vi "Update Test Server.vi"(8 "error in (no error)":errorcluster, 10 "Lines":T2[](array[typedef]) {"OPC UA Data Type" items=["Boolean"=1, "SByte"=2, "Byte"=3, "Int16"=4, "UInt16"=5, "Int32"=6, "UInt32"=7, "Int64"=8, "UInt64"=9, "Float"=10, "Double"=11, "String"=12, "DateTime"=13, "ByteString"=15, "Array of Boolean"=101, "Array of SByte"=102, "Array of Byte"=103, "Array of Int16"=104, "Array of UInt16"=105, "Array of Int32"=106, "Array of UInt32"=107, "Array of Int64"=108, "Array of UInt64"=109, "Array of Float"=110, "Array of Double"=111, "Array of String"=112, "Array of DateTime"=113, "Array of ByteString"=115]}, 11 "OPC UA server refnum in":refnum<k21>) -> (0 "error out":errorcluster, 2 "Server Data":T1(array[cluster]))   [LabVIEW 2013, in "OPC UA Client Tests.lvlib"]
doc: "Forces the OPC UA server to update every line in given configuration. Passes out cluster of node paths and flattened data to be compared to tag bus."
uses:
  OPC UA Client Tests.lvlib
  module/configuration/Line.ctl
  <vilib>/NI/Tag Bus Module Framework/channel/TBM channel.lvclass
  module/configuration/OPC UA Data Type.ctl
  <vilib>/OPCUA/server/Write Bool.vi
  <vilib>/OPCUA/server/Write SByte.vi
  <vilib>/OPCUA/server/Write Byte.vi
  <vilib>/OPCUA/server/Write Int16.vi
  <vilib>/OPCUA/server/Write UInt16.vi
  <vilib>/OPCUA/server/Write Int32.vi
  <vilib>/OPCUA/server/Write UInt32.vi
  <vilib>/OPCUA/server/Write Int64.vi
  <vilib>/OPCUA/server/Write UInt64.vi
  <vilib>/OPCUA/server/Write Float.vi
  <vilib>/OPCUA/server/Write Double.vi
  <vilib>/OPCUA/server/Write String.vi
  <vilib>/OPCUA/server/Write Date Time.vi
  <vilib>/OPCUA/server/Write Byte String.vi
  <vilib>/OPCUA/server/Write Bool Array.vi
  <vilib>/OPCUA/server/Write SByte Array.vi
  <vilib>/OPCUA/server/Write Byte Array.vi
  <vilib>/OPCUA/server/Write Int16 Array.vi
  <vilib>/OPCUA/server/Write UInt16 Array.vi
  <vilib>/OPCUA/server/Write Int32 Array.vi
  <vilib>/OPCUA/server/Write UInt32 Array.vi
  <vilib>/OPCUA/server/Write Int64 Array.vi
  <vilib>/OPCUA/server/Write UInt64 Array.vi
  <vilib>/OPCUA/server/Write Float Array.vi
  <vilib>/OPCUA/server/Write Double Array.vi
  <vilib>/OPCUA/server/Write String Array.vi
  <vilib>/OPCUA/server/Write Date Time Array.vi
  <vilib>/opcua/NI OPC UA Server.lvlib
  module/configuration/OPC UA Client configuration.lvclass
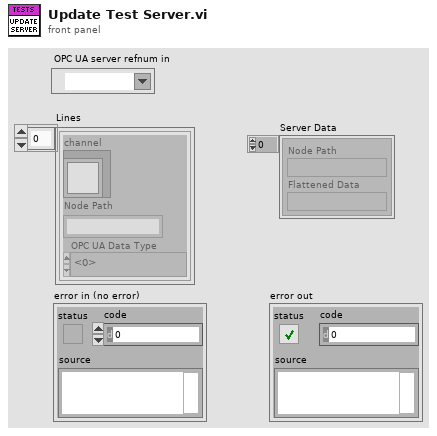
[diagram p1: front panel]
types:
  T1 = cluster{"Node Path":string, "Flattened Data":string}[]
  T2 = typedef "OPC UA Client configuration.lvclass/Line.ctl" = cluster{"channel":refnum<class "TBM channel.lvclass">, "Node Path":string, "OPC UA Data Type":T3}
  T3 = typedef "OPC UA Client configuration.lvclass/OPC UA Data Type.ctl" = u16
  T4 = cluster{"Node Path":string, "Flattened Data":string}
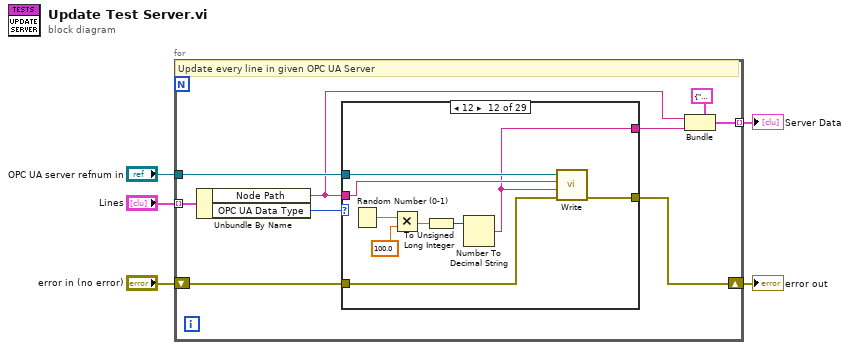
[diagram p0: block diagram]
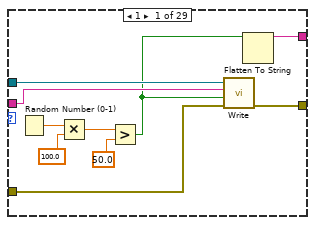
[diagram p2: hidden frame]
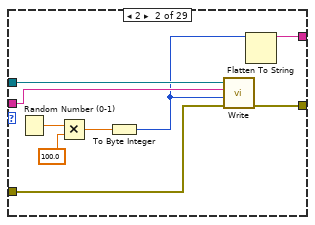
[diagram p3: hidden frame]
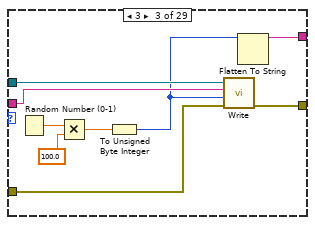
[diagram p4: hidden frame]
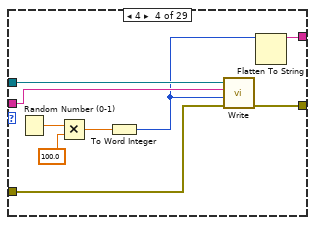
[diagram p5: hidden frame]
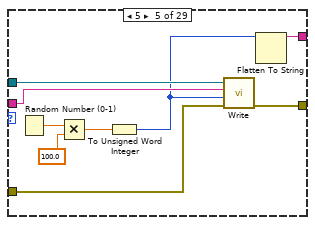
[diagram p6: hidden frame]
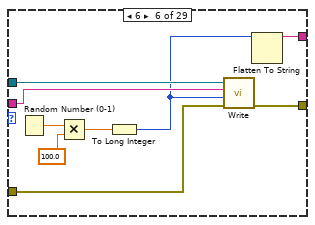
[diagram p7: hidden frame]
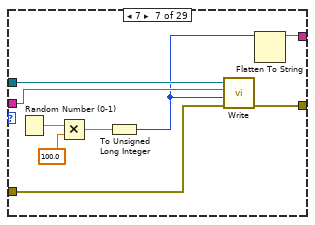
[diagram p8: hidden frame]
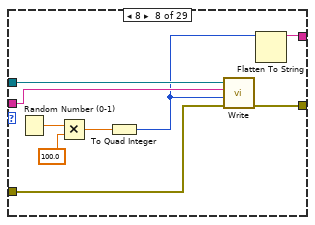
[diagram p9: hidden frame]
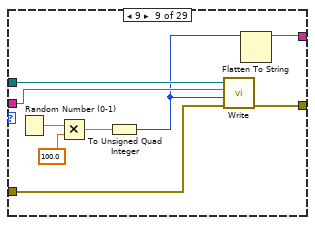
[diagram p10: hidden frame]
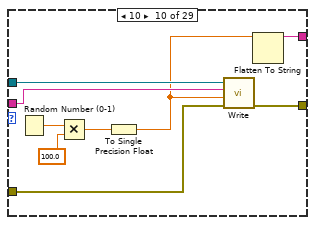
[diagram p11: hidden frame]
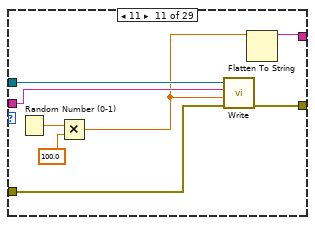
[diagram p12: hidden frame]
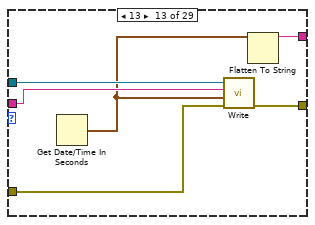
[diagram p13: hidden frame]
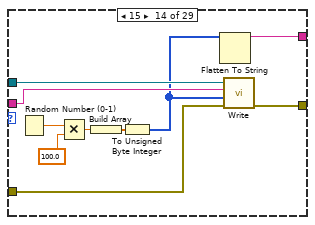
[diagram p14: hidden frame]
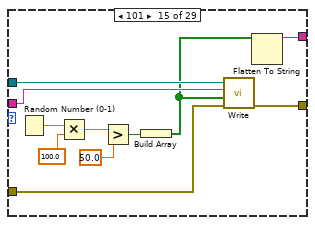
[diagram p15: hidden frame]
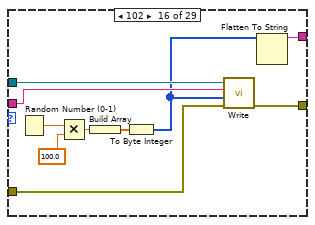
[diagram p16: hidden frame]
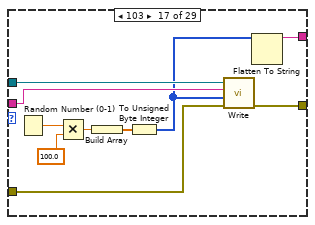
[diagram p17: hidden frame]
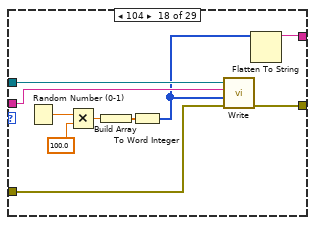
[diagram p18: hidden frame]
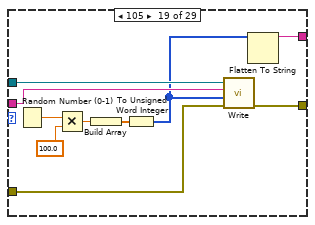
[diagram p19: hidden frame]
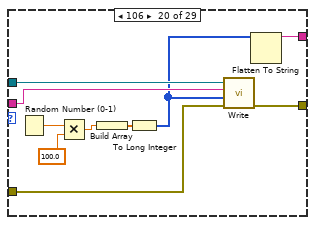
[diagram p20: hidden frame]
diagram:
  n1 = for {
    tunnel: "OPC UA server refnum in" -> [w14]
    tunnel: "Lines" -> [w13] mode=indexing
    tunnel: [w6] -> w1 mode=indexing
    shift-right: [w10] -> w3
    shift-left: "error in (no error)" -> [w11]
    # "Update every line in given OPC UA Server"
    n2 = Unbundle By Name(w13) -> ("Node Path"=w7:string, "OPC UA Data Type"=w12:T3)
    n3 = case shown="12" w12 {
      tunnel: w14 -> [w24 w33 w42 w51 w60 w69 w78 w87 w96 w105 w113 w122 w128 w138 w149 w159 w169 w179 w189 w199 w209 w219 w229 w239 w248 w258 w265 w275 _]
      tunnel: w7 -> [w23 w32 w41 w50 w59 w68 w77 w86 w95 w104 w112 w121 w127 w137 w148 w158 w168 w178 w188 w198 w208 w218 w228 w238 w247 w257 w264 w274 _]
      tunnel: w11 -> [w22 w31 w40 w49 w58 w67 w76 w85 w94 w103 w111 w120 w126 w136 w147 w157 w167 w177 w187 w197 w207 w217 w227 w237 w246 w256 w263 w273 _]
      tunnel: [w21 w30 w39 w48 w57 w66 w75 w84 w93 w102 w110 w119 w125 w135 w146 w156 w166 w176 w186 w196 w206 w216 w226 w236 w245 w255 w262 w272 errorcluster {"status"=TRUE, "code"=0, "source"="Invalid UA Data Type"} ("error out")] -> w10
      tunnel: [w15 w27 w35 w44 w54 w63 w72 w81 w90 w98 w107 w115 w124 w129 w140 w151 w162 w172 w182 w192 w202 w212 w222 w231 w241 w250 w260 w267 "" ("data string")] -> w9
      frame 1 {
        n4 = Random Number (0-1)() -> (number: 0 to 1=w20:dbl)
        n5 = Multiply(x=w20, y=100.0) -> (x*y=w18:dbl)
        n6 = Greater?(x=w18, y=50.0) -> (0:w16:bool)
        n7 = call-poly <vilib>:"Write.vi"("error in (no error)"=w22, "value"=w16, "node path"=w23, "OPC UA server refnum in"=w24) -> ("error out"=w21:errorcluster)  [unwired: 6 in, 1 out]
        n8 = Flatten To String(anything=w16) -> (data string=w15:string)  [unwired: 3 in, 2 out]
      }
      frame 2 {
        n9 = Random Number (0-1)() -> (number: 0 to 1=w29:dbl)
        n10 = Multiply(x=w29, y=100.0) -> (x*y=w26:dbl)
        n11 = To Byte Integer(number=w26) -> (8bit integer=w25:i8)
        n12 = call-poly <vilib>:"Write.vi"("error in (no error)"=w31, "value"=w25, "node path"=w32, "OPC UA server refnum in"=w33) -> ("error out"=w30:errorcluster)  [unwired: 6 in, 1 out]
        n13 = Flatten To String(anything=w25) -> (data string=w27:string)  [unwired: 3 in, 2 out]
      }
      frame 3 {
        n14 = Random Number (0-1)() -> (number: 0 to 1=w38:dbl)
        n15 = Multiply(x=w38, y=100.0) -> (x*y=w36:dbl)
        n16 = To Unsigned Byte Integer(number=w36) -> (unsigned 8bit integer=w34:u8)
        n17 = call-poly <vilib>:"Write.vi"("error in (no error)"=w40, "value"=w34, "node path"=w41, "OPC UA server refnum in"=w42) -> ("error out"=w39:errorcluster)  [unwired: 6 in, 1 out]
        n18 = Flatten To String(anything=w34) -> (data string=w35:string)  [unwired: 3 in, 2 out]
      }
      frame 4 {
        n19 = Random Number (0-1)() -> (number: 0 to 1=w47:dbl)
        n20 = Multiply(x=w47, y=100.0) -> (x*y=w45:dbl)
        n21 = To Word Integer(number=w45) -> (16bit integer=w43:i16)
        n22 = call-poly <vilib>:"Write.vi"("error in (no error)"=w49, "value"=w43, "node path"=w50, "OPC UA server refnum in"=w51) -> ("error out"=w48:errorcluster)  [unwired: 6 in, 1 out]
        n23 = Flatten To String(anything=w43) -> (data string=w44:string)  [unwired: 3 in, 2 out]
      }
      frame 5 {
        n24 = Random Number (0-1)() -> (number: 0 to 1=w56:dbl)
        n25 = Multiply(x=w56, y=100.0) -> (x*y=w53:dbl)
        n26 = To Unsigned Word Integer(number=w53) -> (unsigned 16bit integer=w52:u16)
        n27 = call-poly <vilib>:"Write.vi"("error in (no error)"=w58, "value"=w52, "node path"=w59, "OPC UA server refnum in"=w60) -> ("error out"=w57:errorcluster)  [unwired: 6 in, 1 out]
        n28 = Flatten To String(anything=w52) -> (data string=w54:string)  [unwired: 3 in, 2 out]
      }
      frame 6 {
        n29 = Random Number (0-1)() -> (number: 0 to 1=w65:dbl)
        n30 = Multiply(x=w65, y=100.0) -> (x*y=w62:dbl)
        n31 = To Long Integer(number=w62) -> (32bit integer=w61:i32)
        n32 = call-poly <vilib>:"Write.vi"("error in (no error)"=w67, "value"=w61, "node path"=w68, "OPC UA server refnum in"=w69) -> ("error out"=w66:errorcluster)  [unwired: 6 in, 1 out]
        n33 = Flatten To String(anything=w61) -> (data string=w63:string)  [unwired: 3 in, 2 out]
      }
      frame 7 {
        n34 = Random Number (0-1)() -> (number: 0 to 1=w74:dbl)
        n35 = Multiply(x=w74, y=100.0) -> (x*y=w71:dbl)
        n36 = To Unsigned Long Integer(number=w71) -> (unsigned 32bit integer=w70:u32)
        n37 = call-poly <vilib>:"Write.vi"("error in (no error)"=w76, "value"=w70, "node path"=w77, "OPC UA server refnum in"=w78) -> ("error out"=w75:errorcluster)  [unwired: 6 in, 1 out]
        n38 = Flatten To String(anything=w70) -> (data string=w72:string)  [unwired: 3 in, 2 out]
      }
      frame 8 {
        n39 = Random Number (0-1)() -> (number: 0 to 1=w83:dbl)
        n40 = Multiply(x=w83, y=100.0) -> (x*y=w80:dbl)
        n41 = To Quad Integer(1:w80) -> (0:w79:i64)
        n42 = call-poly <vilib>:"Write.vi"("error in (no error)"=w85, "value"=w79, "node path"=w86, "OPC UA server refnum in"=w87) -> ("error out"=w84:errorcluster)  [unwired: 6 in, 1 out]
        n43 = Flatten To String(anything=w79) -> (data string=w81:string)  [unwired: 3 in, 2 out]
      }
      frame 9 {
        n44 = Random Number (0-1)() -> (number: 0 to 1=w92:dbl)
        n45 = Multiply(x=w92, y=100.0) -> (x*y=w89:dbl)
        n46 = To Unsigned Quad Integer(1:w89) -> (0:w88:u64)
        n47 = call-poly <vilib>:"Write.vi"("error in (no error)"=w94, "value"=w88, "node path"=w95, "OPC UA server refnum in"=w96) -> ("error out"=w93:errorcluster)  [unwired: 6 in, 1 out]
        n48 = Flatten To String(anything=w88) -> (data string=w90:string)  [unwired: 3 in, 2 out]
      }
      frame 10 {
        n49 = Random Number (0-1)() -> (number: 0 to 1=w101:dbl)
        n50 = Multiply(x=w101, y=100.0) -> (x*y=w99:dbl)
        n51 = To Single Precision Float(number=w99) -> (single precision float=w97:sgl)
        n52 = call-poly <vilib>:"Write.vi"("error in (no error)"=w103, "value"=w97, "node path"=w104, "OPC UA server refnum in"=w105) -> ("error out"=w102:errorcluster)  [unwired: 6 in, 1 out]
        n53 = Flatten To String(anything=w97) -> (data string=w98:string)  [unwired: 3 in, 2 out]
      }
      frame 11 {
        n54 = Random Number (0-1)() -> (number: 0 to 1=w109:dbl)
        n55 = Multiply(x=w109, y=100.0) -> (x*y=w106:dbl)
        n56 = call-poly <vilib>:"Write.vi"("error in (no error)"=w111, "value"=w106, "node path"=w112, "OPC UA server refnum in"=w113) -> ("error out"=w110:errorcluster)  [unwired: 6 in, 1 out]
        n57 = Flatten To String(anything=w106) -> (data string=w107:string)  [unwired: 3 in, 2 out]
      }
      frame 12 {
        n58 = Random Number (0-1)() -> (number: 0 to 1=w118:dbl)
        n59 = Multiply(x=w118, y=100.0) -> (x*y=w116:dbl)
        n60 = To Unsigned Long Integer(number=w116) -> (unsigned 32bit integer=w114:u32)
        n61 = Number To Decimal String(number=w114) -> (decimal integer string=w115:string)  [unwired: 1 in]
        n62 = call-poly <vilib>:"Write.vi"("error in (no error)"=w120, "value"=w115, "node path"=w121, "OPC UA server refnum in"=w122) -> ("error out"=w119:errorcluster)  [unwired: 6 in, 1 out]
      }
      frame 13 {
        n63 = Get Date/Time In Seconds() -> (seconds since 1Jan1904=w123:timestamp)
        n64 = call-poly <vilib>:"Write.vi"("error in (no error)"=w126, "value"=w123, "node path"=w127, "OPC UA server refnum in"=w128) -> ("error out"=w125:errorcluster)  [unwired: 6 in, 1 out]
        n65 = Flatten To String(anything=w123) -> (data string=w124:string)  [unwired: 3 in, 2 out]
      }
      frame 15 {
        n66 = Random Number (0-1)() -> (number: 0 to 1=w134:dbl)
        n67 = Multiply(x=w134, y=100.0) -> (x*y=w132:dbl)
        n68 = Build Array(w132) -> (w131:dbl[])
        n69 = To Unsigned Byte Integer(number=w131) -> (unsigned 8bit integer=w130:u8[])
        n70 = Flatten To String(anything=w130) -> (data string=w129:string)  [unwired: 3 in, 2 out]
        n71 = call-poly <vilib>:"Write.vi"("error in (no error)"=w136, "value"=w130, "node path"=w137, "OPC UA server refnum in"=w138) -> ("error out"=w135:errorcluster)  [unwired: 6 in, 1 out]
      }
      frame 101 {
        n72 = Random Number (0-1)() -> (number: 0 to 1=w145:dbl)
        n73 = Multiply(x=w145, y=100.0) -> (x*y=w143:dbl)
        n74 = Greater?(x=w143, y=50.0) -> (0:w141:bool)
        n75 = Build Array(w141) -> (w139:bool[])
        n76 = call-poly <vilib>:"Write.vi"("error in (no error)"=w147, "value"=w139, "node path"=w148, "OPC UA server refnum in"=w149) -> ("error out"=w146:errorcluster)  [unwired: 6 in, 1 out]
        n77 = Flatten To String(anything=w139) -> (data string=w140:string)  [unwired: 3 in, 2 out]
      }
      frame 102 {
        n78 = Random Number (0-1)() -> (number: 0 to 1=w155:dbl)
        n79 = Multiply(x=w155, y=100.0) -> (x*y=w153:dbl)
        n80 = Build Array(w153) -> (w152:dbl[])
        n81 = To Byte Integer(number=w152) -> (8bit integer=w150:i8[])
        n82 = call-poly <vilib>:"Write.vi"("error in (no error)"=w157, "value"=w150, "node path"=w158, "OPC UA server refnum in"=w159) -> ("error out"=w156:errorcluster)  [unwired: 6 in, 1 out]
        n83 = Flatten To String(anything=w150) -> (data string=w151:string)  [unwired: 3 in, 2 out]
      }
      frame 103 {
        n84 = Random Number (0-1)() -> (number: 0 to 1=w165:dbl)
        n85 = Multiply(x=w165, y=100.0) -> (x*y=w163:dbl)
        n86 = Build Array(w163) -> (w161:dbl[])
        n87 = To Unsigned Byte Integer(number=w161) -> (unsigned 8bit integer=w160:u8[])
        n88 = call-poly <vilib>:"Write.vi"("error in (no error)"=w167, "value"=w160, "node path"=w168, "OPC UA server refnum in"=w169) -> ("error out"=w166:errorcluster)  [unwired: 6 in, 1 out]
        n89 = Flatten To String(anything=w160) -> (data string=w162:string)  [unwired: 3 in, 2 out]
      }
      frame 104 {
        n90 = Random Number (0-1)() -> (number: 0 to 1=w175:dbl)
        n91 = Multiply(x=w175, y=100.0) -> (x*y=w173:dbl)
        n92 = Build Array(w173) -> (w171:dbl[])
        n93 = To Word Integer(number=w171) -> (16bit integer=w170:i16[])
        n94 = call-poly <vilib>:"Write.vi"("error in (no error)"=w177, "value"=w170, "node path"=w178, "OPC UA server refnum in"=w179) -> ("error out"=w176:errorcluster)  [unwired: 6 in, 1 out]
        n95 = Flatten To String(anything=w170) -> (data string=w172:string)  [unwired: 3 in, 2 out]
      }
      frame 105 {
        n96 = Random Number (0-1)() -> (number: 0 to 1=w185:dbl)
        n97 = Multiply(x=w185, y=100.0) -> (x*y=w183:dbl)
        n98 = Build Array(w183) -> (w181:dbl[])
        n99 = To Unsigned Word Integer(number=w181) -> (unsigned 16bit integer=w180:u16[])
        n100 = call-poly <vilib>:"Write.vi"("error in (no error)"=w187, "value"=w180, "node path"=w188, "OPC UA server refnum in"=w189) -> ("error out"=w186:errorcluster)  [unwired: 6 in, 1 out]
        n101 = Flatten To String(anything=w180) -> (data string=w182:string)  [unwired: 3 in, 2 out]
      }
      frame 106 {
        n102 = Random Number (0-1)() -> (number: 0 to 1=w195:dbl)
        n103 = Multiply(x=w195, y=100.0) -> (x*y=w193:dbl)
        n104 = Build Array(w193) -> (w191:dbl[])
        n105 = To Long Integer(number=w191) -> (32bit integer=w190:i32[])
        n106 = call-poly <vilib>:"Write.vi"("error in (no error)"=w197, "value"=w190, "node path"=w198, "OPC UA server refnum in"=w199) -> ("error out"=w196:errorcluster)  [unwired: 6 in, 1 out]
        n107 = Flatten To String(anything=w190) -> (data string=w192:string)  [unwired: 3 in, 2 out]
      }
      frame 107 {
        n108 = Random Number (0-1)() -> (number: 0 to 1=w205:dbl)
        n109 = Multiply(x=w205, y=100.0) -> (x*y=w203:dbl)
        n110 = Build Array(w203) -> (w201:dbl[])
        n111 = To Unsigned Long Integer(number=w201) -> (unsigned 32bit integer=w200:u32[])
        n112 = call-poly <vilib>:"Write.vi"("error in (no error)"=w207, "value"=w200, "node path"=w208, "OPC UA server refnum in"=w209) -> ("error out"=w206:errorcluster)  [unwired: 6 in, 1 out]
        n113 = Flatten To String(anything=w200) -> (data string=w202:string)  [unwired: 3 in, 2 out]
      }
      frame 108 {
        n114 = Random Number (0-1)() -> (number: 0 to 1=w215:dbl)
        n115 = Multiply(x=w215, y=100.0) -> (x*y=w213:dbl)
        n116 = Build Array(w213) -> (w211:dbl[])
        n117 = To Quad Integer(1:w211) -> (0:w210:i64[])
        n118 = call-poly <vilib>:"Write.vi"("error in (no error)"=w217, "value"=w210, "node path"=w218, "OPC UA server refnum in"=w219) -> ("error out"=w216:errorcluster)  [unwired: 6 in, 1 out]
        n119 = Flatten To String(anything=w210) -> (data string=w212:string)  [unwired: 3 in, 2 out]
      }
      frame 109 {
        n120 = Random Number (0-1)() -> (number: 0 to 1=w225:dbl)
        n121 = Multiply(x=w225, y=100.0) -> (x*y=w223:dbl)
        n122 = Build Array(w223) -> (w221:dbl[])
        n123 = To Unsigned Quad Integer(1:w221) -> (0:w220:u64[])
        n124 = call-poly <vilib>:"Write.vi"("error in (no error)"=w227, "value"=w220, "node path"=w228, "OPC UA server refnum in"=w229) -> ("error out"=w226:errorcluster)  [unwired: 6 in, 1 out]
        n125 = Flatten To String(anything=w220) -> (data string=w222:string)  [unwired: 3 in, 2 out]
      }
      frame 110 {
        n126 = Random Number (0-1)() -> (number: 0 to 1=w235:dbl)
        n127 = Multiply(x=w235, y=100.0) -> (x*y=w233:dbl)
        n128 = Build Array(w233) -> (w232:dbl[])
        n129 = To Single Precision Float(number=w232) -> (single precision float=w230:sgl[])
        n130 = call-poly <vilib>:"Write.vi"("error in (no error)"=w237, "value"=w230, "node path"=w238, "OPC UA server refnum in"=w239) -> ("error out"=w236:errorcluster)  [unwired: 6 in, 1 out]
        n131 = Flatten To String(anything=w230) -> (data string=w231:string)  [unwired: 3 in, 2 out]
      }
      frame 111 {
        n132 = Random Number (0-1)() -> (number: 0 to 1=w244:dbl)
        n133 = Multiply(x=w244, y=100.0) -> (x*y=w242:dbl)
        n134 = Build Array(w242) -> (w240:dbl[])
        n135 = call-poly <vilib>:"Write.vi"("error in (no error)"=w246, "value"=w240, "node path"=w247, "OPC UA server refnum in"=w248) -> ("error out"=w245:errorcluster)  [unwired: 6 in, 1 out]
        n136 = Flatten To String(anything=w240) -> (data string=w241:string)  [unwired: 3 in, 2 out]
      }
      frame 112 {
        n137 = Random Number (0-1)() -> (number: 0 to 1=w254:dbl)
        n138 = Multiply(x=w254, y=100.0) -> (x*y=w252:dbl)
        n139 = Number To Decimal String(number=w252) -> (decimal integer string=w251:string)  [unwired: 1 in]
        n140 = Build Array(w251) -> (w249:string[])
        n141 = call-poly <vilib>:"Write.vi"("error in (no error)"=w256, "value"=w249, "node path"=w257, "OPC UA server refnum in"=w258) -> ("error out"=w255:errorcluster)  [unwired: 6 in, 1 out]
        n142 = Flatten To String(anything=w249) -> (data string=w250:string)  [unwired: 3 in, 2 out]
      }
      frame 113 {
        n143 = Get Date/Time In Seconds() -> (seconds since 1Jan1904=w261:timestamp)
        n144 = Build Array(w261) -> (w259:timestamp[])
        n145 = call-poly <vilib>:"Write.vi"("error in (no error)"=w263, "value"=w259, "node path"=w264, "OPC UA server refnum in"=w265) -> ("error out"=w262:errorcluster)  [unwired: 6 in, 1 out]
        n146 = Flatten To String(anything=w259) -> (data string=w260:string)  [unwired: 3 in, 2 out]
      }
      frame 115 {
        n147 = Random Number (0-1)() -> (number: 0 to 1=w271:dbl)
        n148 = Multiply(x=w271, y=100.0) -> (x*y=w269:dbl)
        n149 = Number To Decimal String(number=w269) -> (decimal integer string=w268:string)  [unwired: 1 in]
        n150 = Build Array(w268) -> (w266:string[])
        n151 = call-poly <vilib>:"Write.vi"("error in (no error)"=w273, "value"=w266, "node path"=w274, "OPC UA server refnum in"=w275) -> ("error out"=w272:errorcluster)  [unwired: 6 in, 1 out]
        n152 = Flatten To String(anything=w266) -> (data string=w267:string)  [unwired: 3 in, 2 out]
      }
      frame 0, Default {
      }
    }
    n153 = Bundle(cluster=T4 {"Node Path"="", "Flattened Data"=""}, "Node Path"=w7, "Flattened Data"=w9) -> (w6:T4)
  }
  "error out" <- w3
  "Server Data" <- w1
